vi "Get_Rig_Preferences.vi"(1 "EnFlo_Data_Folder_Setup":T1="EnFlo_Data on Server", 2 "Rig Setup":string) -> ()   [LabVIEW 2011]
uses:
  Anemometry/Anemometry Sub Vis/Controls/EnFlo_Data_Folder_Setup.ctl
  Anemometry/Anemometry Sub Vis/Globals/Constants_global.vi
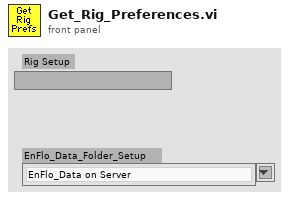
[diagram p1: front panel]
types:
  T1 = typedef "EnFlo_Data_Folder_Setup.ctl" = string
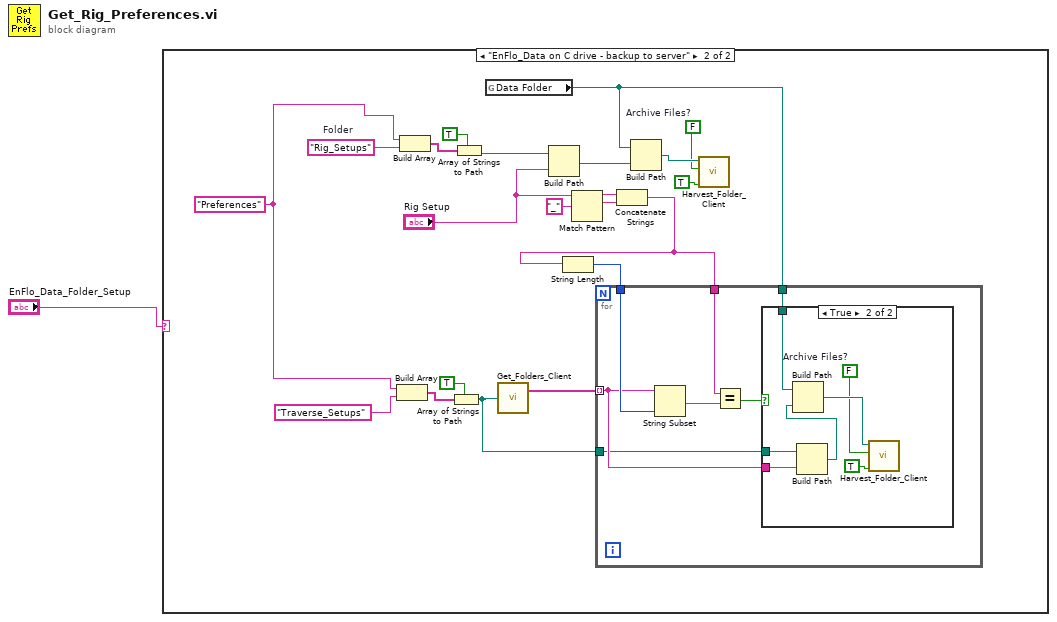
[diagram p0: block diagram]
diagram:
  n1 = case shown="\"EnFlo_Data on C drive - backup to server\"" "EnFlo_Data_Folder_Setup" {
    frame "False", Default {
    }
    frame "EnFlo_Data on C drive - backup to server" {
      w2 = FALSE  # Archive Files?
      w17 = "Rig_Setups"  # Folder
      w16 = "Preferences" ("name or relative path")
      n2 = Build Array(w16, "Traverse_Setups" ("name or relative path")) -> (w22:string[])
      n3 = Build Array(w16, w17) -> (w18:string[])
      n4 = Array of Strings to Path(0:w22, 1:TRUE ("relative")) -> (2:w11:path)
      n5 = Array of Strings to Path(0:w18, 1:TRUE ("relative")) -> (2:w14:path)
      n6 = global read "Constants_global.vi" "Data Folder"() -> (w8:path)
      n7 = call "Get_Folders_Client.vi"("Relative Path"=w11) -> ("Folder Names"=w13:string[])  [unwired: 1 out]
      n8 = Build Path(base path=w14, name or relative path="Rig Setup") -> (appended path=w10:path)
      n9 = Match Pattern(string="Rig Setup", regular expression="_") -> (before substring=w5:string, match substring=w4:string)  [unwired: 1 in, 2 out]
      n10 = Concatenate Strings(w5, w4) -> (w3:string)
      n11 = String Length(string=w3) -> (length=w12:i32)
      n12 = for {
        tunnel: w13 -> [w25] mode=indexing
        tunnel: w12 -> [w29]
        tunnel: w3 -> [w27]
        tunnel: w11 -> [w24]
        tunnel: w8 -> [w23]
        n13 = String Subset(string=w25, length (rest)=w29) -> (substring=w28:string)  [unwired: 1 in]
        n14 = Equal?(x=w27, y=w28) -> (x = y?=w26:bool)
        n15 = case shown="True" w26 {
          tunnel: w25 -> [_ w35]
          tunnel: w24 -> [_ w31]
          tunnel: w23 -> [_ w34]
          frame False {
          }
          frame True {
            w30 = FALSE  # Archive Files?
            n16 = Build Path(base path=w31, name or relative path=w35) -> (appended path=w33:path)
            n17 = Build Path(base path=w34, name or relative path=w33) -> (appended path=w32:path)
            n18 = call "Harvest_Folder_Client.vi"("Get all Server Files"=TRUE, "Archive Files?"=w30, "Folder to Harvest"=w32) -> ()  [unwired: 1 in, 2 out]
          }
        }
      }
      n19 = Build Path(base path=w8, name or relative path=w10) -> (appended path=w9:path)
      n20 = call "Harvest_Folder_Client.vi"("Get all Server Files"=TRUE, "Archive Files?"=w2, "Folder to Harvest"=w9) -> ()  [unwired: 1 in, 2 out]
    }
  }
